vi "Wait For Bytes.vi"(7 "Timeout (100 ms)":u32=100, 8 "Error In":errorcluster, 10 "Num Bytes":u32, 11 "LINX Device Config":T1) -> (0 "Error Out":errorcluster, 1 "Timeout":bool, 2 "Num Bytes":u32, 3 "LINX Device Config":T1)   [LabVIEW 2020, in "LMH-LINX.lvlib" / "Device.lvlib"]
doc: "Wait until the specified number of bytes are abailable at the serial port or a timeout occurs."
uses:
  Device.lvlib
  Type Defs/LINX Device Config.ctl
  Type Defs/Interface.ctl
  Type Defs/TCP Config.ctl
  Type Defs/Channels.ctl
  LMH-LINX.lvlib
panel:
  out "Numeric Control":i32
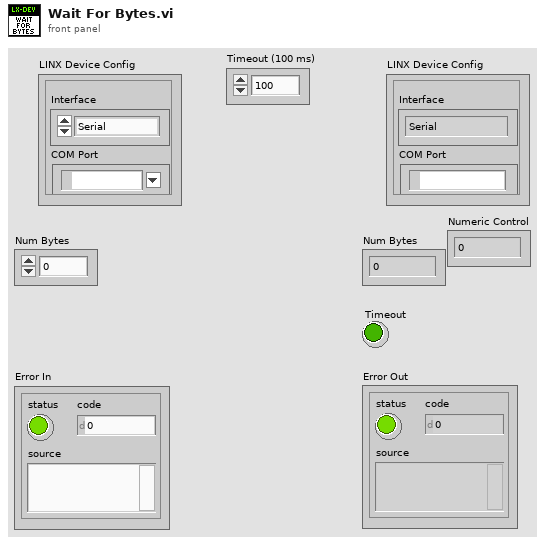
[diagram p1: front panel]
types:
  T1 = typedef "LMH-LINX.lvlib/Device.lvlib/LINX Device Config.ctl" = cluster{"Interface":T2, "COM Port":refnum<visa-resource-name>, "TCP Configuration":T3, "Device Family":u8, "Device ID":u8, "Device Name":string, "TCP Ref":refnum<k5>, "Channels":T4}
  T2 = typedef "LMH-LINX.lvlib/Interface.ctl" = enum16{"Serial", "TCP"}
  T3 = typedef "LMH-LINX.lvlib/Device.lvlib/TCP Config.ctl" = cluster{"IP Address":string, "Port":u16}
  T4 = typedef "LMH-LINX.lvlib/Channels.ctl" = cluster{"DI":u8[], "DO":u8[], "AI":u8[], "AO":u8[], "PWM":u8[], "QE":u8[], "UART":u8[], "I2C 2":u8[], "SPI":u8[], "CAN":u8[], "Servo":u8[], "AI Ref (V)":dbl, "AI Resolution (Bits)":u8, "AO Ref (V)":dbl, "AO Resolution (Bits)":u8}
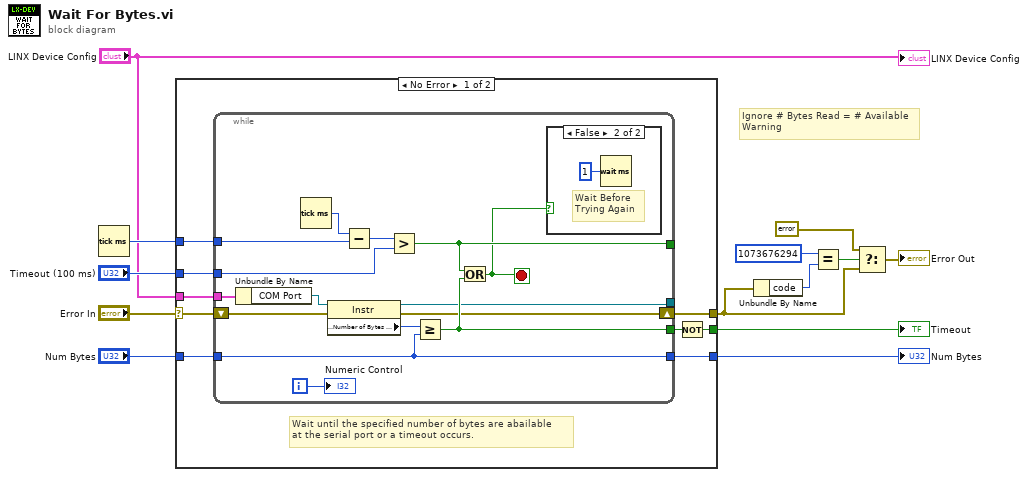
[diagram p0: block diagram]
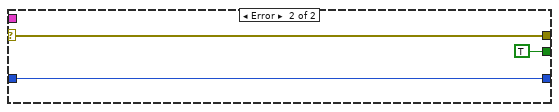
[diagram p3: hidden frame]
diagram:
  # "Ignore # Bytes Read = # Available\nWarning"
  n1 = Tick Count (ms)() -> (millisecond timer value=w12:u32)
  n2 = case shown="No Error" "Error In" {
    selector: "Error In" -> [w16 w41]
    tunnel: [w22 w41] -> w6
    tunnel: "LINX Device Config" -> [w21 _]
    tunnel: "Timeout (100 ms)" -> [w20 _]
    tunnel: w12 -> [w19 _]
    tunnel: [w14 TRUE] -> w7
    tunnel: "Num Bytes" -> [w18 w40]
    tunnel: [w17 w40] -> w10
    frame No Error {
      # "Wait until the specified number of bytes are abailable\nat the serial port or a timeout occurs."
      n3 = while {
        tunnel: w19 -> [w36]
        tunnel: w20 -> [w34]
        tunnel: w21 -> [w26]
        shift-right: [w29] -> w22
        shift-left: w16 -> [w33]
        tunnel: [w30] -> w15
        tunnel: [w31] -> _
        tunnel: [w28] -> _
        tunnel: w18 -> [w27]
        tunnel: [w27] -> w17
        i -> [w23]
        stop <- w24 stop-if-true
        n4 = Unbundle By Name(w26) -> ("COM Port"=w25:refnum<visa-resource-name>)
        n5 = Tick Count (ms)() -> (millisecond timer value=w37:u32)
        n6 = property class="Instr"(reference=w25, error in=w33) -> (reference out=w28:refnum<visa-resource-name>, error out=w29:errorcluster, "Serial Settings:Number of Bytes at Serial Port"=w32:u32)
        n7 = Subtract(x=w37, y=w36) -> (x-y=w35:u32)
        n8 = Greater?(x=w35, y=w34) -> (0:w31:bool)
        n9 = Greater Or Equal?(x=w32, y=w27) -> (x >= y?=w30:bool)
        n10 = Or(x=w31, y=w30) -> (x .or. y?=w24:bool)
        n11 = case shown="False" w24 {
          frame True {
          }
          frame False {
            # "Wait Before\nTrying Again"
            n12 = Wait (ms)(milliseconds to wait=u32 1) -> ()  [unwired: 1 out]
          }
        }
        "Numeric Control" <- w23
      }
      n13 = Not(x=w15) -> (.not. x?=w14:bool)
    }
    frame Error {
    }
  }
  "Timeout" <- w7
  "Num Bytes" <- w10
  n14 = Unbundle By Name(w6) -> ("code"=w5:i32)
  n15 = Equal?(x=1073676294, y=w5) -> (x = y?=w3:bool)
  n16 = Select(t=errorcluster {"status"=FALSE, "code"=0, "source"=""}, s=w3, f=w6) -> (s? t:f=→"Error Out":errorcluster)
  "LINX Device Config" <- "LINX Device Config"
